vi "Update Build Version.vi"(8 "error in (no error)":errorcluster, 11 "PostBuildSupport in":refnum<class "PostBuildSupport.lvclass">) -> (0 "error out":errorcluster, 3 "PostBuildSupport out":refnum<class "PostBuildSupport.lvclass">)   [LabVIEW 2016, in "PostBuildSupport.lvclass"]
uses:
  PostBuildSupport.lvclass
  <vilib>/AppBuilder/AB_API_Simple/Build Specification Version.ctl
  PostBuildSupport.lvclass/PostBuildSupport.ctl
  <vilib>/AppBuilder/AB_API_Simple/Set Build Specification Version (path).vi
  <vilib>/AppBuilder/AB_API_Simple/NI_App_Builder_API.lvlib
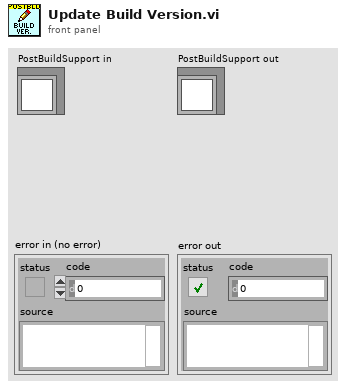
[diagram p1: front panel]
types:
  T1 = typedef "NI_App_Builder_API.lvlib/Build Specification Version.ctl" = cluster{"Major":u16, "Minor":u16, "Fix":u16, "Build":u16}
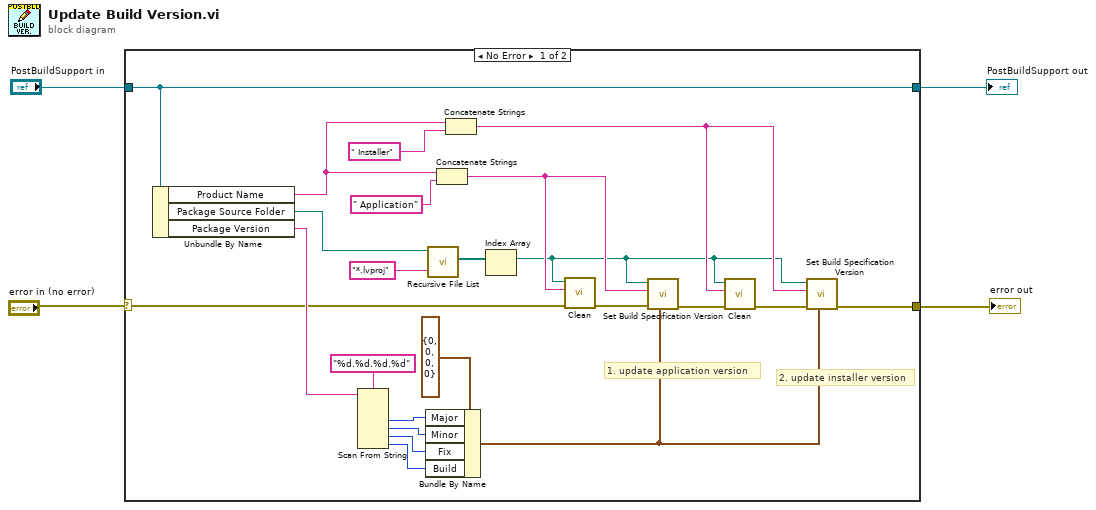
[diagram p0: block diagram]
diagram:
  n1 = case shown="No Error" "error in (no error)" {
    selector: "error in (no error)" -> [w5 w28]
    tunnel: [w27 w28] -> w4
    tunnel: "PostBuildSupport in" -> [w6 w29]
    tunnel: [w6 w29] -> w2
    frame No Error {
      # "2. update installer version"
      # "1. update application version"
      n2 = Unbundle By Name(w6) -> ("Product Name"=w8:string, "Package Source Folder"=w9:path, "Package Version"=w7:string)
      n3 = Scan From String(format string="%d.%d.%d.%d", input string=w7) -> (output 1=w22:i32, output 2=w25:i32, output 3=w21:i32, output 4=w24:i32)  [unwired: 6 in, 3 out]
      n4 = Bundle By Name(cluster=T1 {"Major"=0, "Minor"=0, "Fix"=0, "Build"=0} ("Build Specification Version"), "Major"=w22, "Minor"=w25, "Fix"=w21, "Build"=w24) -> (w26:T1)
      n5 = call <vilib>:"Recursive File List.vi"("pattern"="*.lvproj", "Folder Path"=w9) -> ("All Files in Dir"=w11:path[])  [unwired: 5 in, 4 out]
      n6 = Concatenate Strings(w8, " Application" ("Name of target (My Computer)")) -> (w15:string)
      n7 = Concatenate Strings(w8, " Installer" ("Name of target (My Computer)")) -> (w13:string)
      n8 = Index Array(array=w11) -> (element=w10:path)  [unwired: 1 in]
      n9 = call <vilib>:"Clean.vi"("error in (no error)"=w5, "Name of build specification (if empty: clean all)"=w15, "Path to project"=w10) -> ("error out"=w19:errorcluster)  [unwired: 8 in]
      n10 = call-poly <vilib>:"Set Build Specification Version.vi"("Build Specification Version"=w26, "error in (no error)"=w19, "Name of build specification"=w15, "Path to project"=w10) -> ("error out"=w18:errorcluster)  [unwired: 7 in]
      n11 = call <vilib>:"Clean.vi"("error in (no error)"=w18, "Name of build specification (if empty: clean all)"=w13, "Path to project"=w10) -> ("error out"=w17:errorcluster)  [unwired: 8 in]
      n12 = call-poly <vilib>:"Set Build Specification Version.vi"("Build Specification Version"=w26, "error in (no error)"=w17, "Name of build specification"=w13, "Path to project"=w10) -> ("error out"=w27:errorcluster)  [unwired: 7 in]
    }
    frame Error {
    }
  }
  "error out" <- w4
  "PostBuildSupport out" <- w2
